vi "Write (DBL).vi"(9 "error in (no error)":errorcluster, 10 "DBL Value":dbl, 11 "Config Element in":refnum<class "Config Element.lvclass">) -> (1 "error out":errorcluster, 3 "Config Element out":refnum<class "Config Element.lvclass">)   [LabVIEW 2023, in "CDM-Config.lvlib" / "Config Element.lvclass"]
uses:
  Config Element.lvclass
  Value Type.ctl
  Config Element.lvclass/Config Element.ctl
  CDM-Config.lvlib
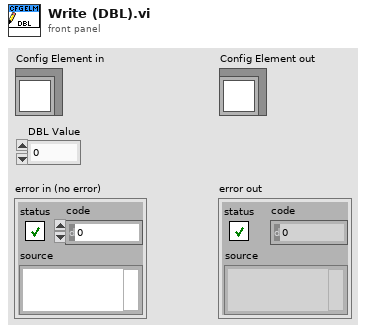
[diagram p1: front panel]
types:
  T1 = typedef "CDM-Config.lvlib/Value Type.ctl" = enum16{"String", "Number", "Bool", "Object", "Array"}
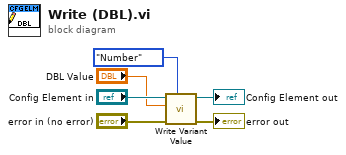
[diagram p0: block diagram]
diagram:
  n1 = call "Write Variant Value.vi"("Value Type"=Value_Type."Number", "error in (no error)"="error in (no error)", "Value"="DBL Value", "Config Element in"="Config Element in") -> ("error out"=→"error out":errorcluster, "Config Element out"=→"Config Element out":refnum<class "Config Element.lvclass">)  [unwired: 6 in]
